vi "get_data.vi"(0 "Image in":refnum<class "Image.lvclass">, 11 "error in (no error)":errorcluster) -> (1 "Image Pixels (U8)":u8[][](array[numeric]), 3 "Image Pixels (I16)":i16[][](array[numeric]), 4 "Image out":refnum<class "Image.lvclass">, 6 "Image Pixels (Float)":sgl[][](array[numeric]), 8 "Image Pixels (U16)":u16[][](array[numeric]), 10 "Image Pixels (U32)":u32[][](array[numeric]), 12 "Image Type":T1 items=["Grayscale (U8)", "Grayscale (I16)", "Grayscale (SGL)", "Complex (CSG)", "RGB (U32)", "HSL (U32)", "RGB (U64)"], 14 "Image Pixels (U64)":T2[][](array[typedef]), 15 "error out":errorcluster)   [LabVIEW 2010, in "Image.lvclass"]
uses:
  Image.lvclass
  storage_mode.ctl
  error_codes_ring.ctl
  ErrorController/ErrorController/class_data.vi
  ErrorController/ErrorController/ErrorController.lvclass
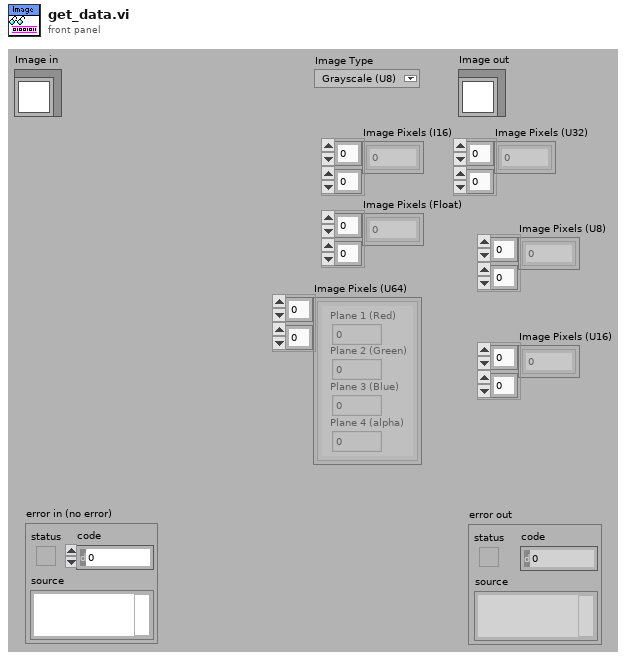
[diagram p1: front panel]
types:
  T1 = typedef "Image Type" = u32
  T2 = typedef "Color (U64)" = cluster{"Plane 3 (Blue)":u16, "Plane 2 (Green)":u16, "Plane 1 (Red)":u16, "Plane 4 (alpha)":u16}
  T3 = typedef "Image.lvclass/storage_mode.ctl" = enum16{"RAM", "disk"}
  T4 = typedef "IMAQ Image.ctl" = refnum<image>
  T5 = typedef "Image.lvclass/error_codes_ring.ctl" = u16
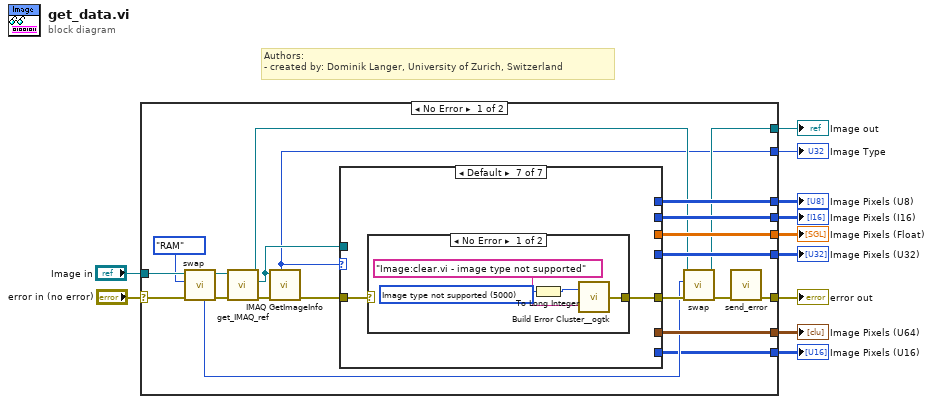
[diagram p0: block diagram]
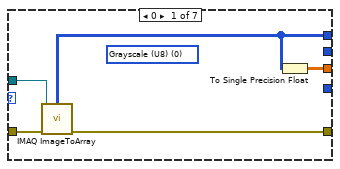
[diagram p2: hidden frame]
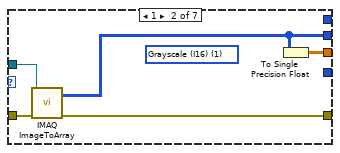
[diagram p3: hidden frame]
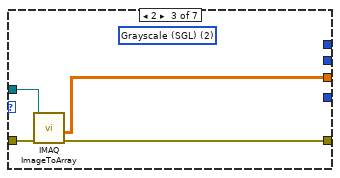
[diagram p4: hidden frame]
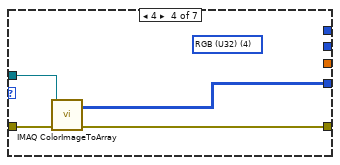
[diagram p5: hidden frame]
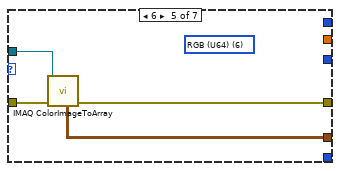
[diagram p6: hidden frame]
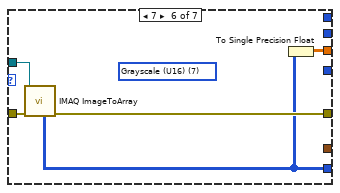
[diagram p7: hidden frame]
diagram:
  # "Authors: \n- created by: Dominik Langer, University of Zurich, Switzerland"
  n1 = case shown="No Error" "error in (no error)" {
    selector: "error in (no error)" -> [w24 w68]
    tunnel: [w12 w68] -> w10
    tunnel: [w18 w67] -> w8
    tunnel: "Image in" -> [w23 w67]
    tunnel: [w29 _] -> w7
    tunnel: [w28 _] -> w6
    tunnel: [w27 _] -> w5
    tunnel: [w26 _] -> w4
    tunnel: [w25 _] -> w3
    tunnel: [w14 _] -> w2
    tunnel: [w15 _] -> w1
    frame No Error {
      n2 = call-dynamic "swap.vi"("error in (no error)"=w24, "storage type target"=storage_mode."RAM", "Image in"=w23) -> ("error out"=w21:errorcluster, "Image out"=w22:refnum<class "Image.lvclass">, "previous storage mode"=w16:T3)  [unwired: 6 out]
      n3 = call-dynamic "get_IMAQ_ref.vi"("error in (no error)"=w21, "Image.lvclass in"=w22) -> ("error out"=w32:errorcluster, "Image"=w30:T4, "Image.lvclass out"=w19:refnum<class "Image.lvclass">)  [unwired: 7 out]
      n4 = call "IMAQ GetImageInfo"("error in (no error)"=w32, "Image"=w30) -> ("error out"=w31:errorcluster, "Image Type"=w14:T1)  [unwired: 8 out]
      n5 = case shown="Default" w14 {
        tunnel: w31 -> [w37 w42 w46 w50 w54 w59 w61]
        tunnel: w30 -> [w36 w40 w45 w49 w52 w57 _]
        tunnel: [w35 w41 w44 w47 w53 w58 w60] -> w17
        tunnel: [w33 _ _ _ _ _ _] -> w29
        tunnel: [_ w38 _ _ _ _ _] -> w28
        tunnel: [w34 w39 w43 _ _ w56 _] -> w27
        tunnel: [_ _ _ w48 _ _ _] -> w26
        tunnel: [_ _ _ _ w51 _ _] -> w25
        tunnel: [_ _ _ _ _ w55 _] -> w15
        frame 0 {
          (unwired) T1 0 items=["Grayscale (U8)", "Grayscale (I16)", "Grayscale (SGL)", "Complex (CSG)", "RGB (U32)", "HSL (U32)", "RGB (U64)", "Grayscale (U16)"] ("Image Type")
          n6 = call "IMAQ ImageToArray"("error in (no error)"=w37, "Image"=w36) -> ("error out"=w35:errorcluster, "Image Pixels (U8)"=w33:u8[][])  [unwired: 1 in, 4 out]
          n7 = To Single Precision Float(number=w33) -> (single precision float=w34:sgl[][])
        }
        frame 1 {
          (unwired) T1 1 items=["Grayscale (U8)", "Grayscale (I16)", "Grayscale (SGL)", "Complex (CSG)", "RGB (U32)", "HSL (U32)", "RGB (U64)", "Grayscale (U16)"] ("Image Type")
          n8 = call "IMAQ ImageToArray"("error in (no error)"=w42, "Image"=w40) -> ("error out"=w41:errorcluster, "Image Pixels (I16)"=w38:i16[][])  [unwired: 1 in, 4 out]
          n9 = To Single Precision Float(number=w38) -> (single precision float=w39:sgl[][])
        }
        frame 2 {
          (unwired) T1 2 items=["Grayscale (U8)", "Grayscale (I16)", "Grayscale (SGL)", "Complex (CSG)", "RGB (U32)", "HSL (U32)", "RGB (U64)", "Grayscale (U16)"] ("Image Type")
          n10 = call "IMAQ ImageToArray"("error in (no error)"=w46, "Image"=w45) -> ("Image Pixels (Float)"=w43:sgl[][], "error out"=w44:errorcluster)  [unwired: 1 in, 4 out]
        }
        frame 4 {
          (unwired) T1 4 items=["Grayscale (U8)", "Grayscale (I16)", "Grayscale (SGL)", "Complex (CSG)", "RGB (U32)", "HSL (U32)", "RGB (U64)", "Grayscale (U16)"] ("Image Type")
          n11 = call "IMAQ ColorImageToArray"("Image"=w49, "error in (no error)"=w50) -> ("Image Pixels (U32)"=w48:u32[][], "error out"=w47:errorcluster)  [unwired: 1 in, 2 out]
        }
        frame 6 {
          (unwired) T1 6 items=["Grayscale (U8)", "Grayscale (I16)", "Grayscale (SGL)", "Complex (CSG)", "RGB (U32)", "HSL (U32)", "RGB (U64)", "Grayscale (U16)"] ("Image Type")
          n12 = call "IMAQ ColorImageToArray"("Image"=w52, "error in (no error)"=w54) -> ("error out"=w53:errorcluster, "Image Pixels (U64)"=w51:T2[][])  [unwired: 1 in, 2 out]
        }
        frame 7 {
          (unwired) T1 7 items=["Grayscale (U8)", "Grayscale (I16)", "Grayscale (SGL)", "Complex (CSG)", "RGB (U32)", "HSL (U32)", "RGB (U64)", "Grayscale (U16)"] ("Image Type")
          n13 = call "IMAQ ImageToArray"("error in (no error)"=w59, "Image"=w57) -> ("Image Pixels (U16)"=w55:u16[][], "error out"=w58:errorcluster)  [unwired: 1 in, 4 out]
          n14 = To Single Precision Float(number=w55) -> (single precision float=w56:sgl[][])
        }
        frame Default {
          n15 = case shown="No Error" w61 {
            selector: w61 -> [_ w66]
            tunnel: [w65 w66] -> w60
            frame No Error {
              w63 = T5 5000 items=["Image type not supported"=5000] ("Ring")
              n16 = To Long Integer(number=w63) -> (32bit integer=w62:i32)
              n17 = call <userlib>:"Build Error Cluster__ogtk.vi"("String to Prepend to source (\"\")"="Image:clear.vi - image type not supported" ("String to Prepend to source (\"\")"), "code"=w62) -> ("error out"=w65:errorcluster)
            }
            frame Error {
            }
          }
        }
      }
      n18 = call-dynamic "swap.vi"("error in (no error)"=w17, "storage type target"=w16, "Image in"=w19) -> ("error out"=w13:errorcluster, "Image out"=w18:refnum<class "Image.lvclass">)  [unwired: 7 out]
      n19 = call "send_error.vi"("error in (no error)"=w13) -> ("error out"=w12:errorcluster)  [unwired: 10 in]
    }
    frame Error {
    }
  }
  "error out" <- w10
  "Image out" <- w8
  "Image Pixels (U8)" <- w7
  "Image Pixels (I16)" <- w6
  "Image Pixels (Float)" <- w5
  "Image Pixels (U32)" <- w4
  "Image Pixels (U64)" <- w3
  "Image Type" <- w2
  "Image Pixels (U16)" <- w1
